vi "MultiPlotting_6PlotForADC.vi"(0 "2D-DataIn":dbl[][](array[numeric]), 3 "DisplayControl":T2 {"Scale" items=["L", "R"]; "Y - axes"."Y 6" items=["", "Realtime_sec", "Intervaltime_sec", "OscillatorFreq_Hz", "SR7265_1_Vx_Volt", "SR7265_1_Vy_Volt", "Ohm"]; "Y - axes"."Y 5" items=["", "Realtime_sec", "Intervaltime_sec", "OscillatorFreq_Hz", "SR7265_1_Vx_Volt", "SR7265_1_Vy_Volt", "Ohm"]; "Y - axes"."Y 4" items=["", "Realtime_sec", "Intervaltime_sec", "OscillatorFreq_Hz", "SR7265_1_Vx_Volt", "SR7265_1_Vy_Volt", "Ohm"]; "Y - axes"."Y 3" items=["", "Realtime_sec", "Intervaltime_sec", "OscillatorFreq_Hz", "SR7265_1_Vx_Volt", "SR7265_1_Vy_Volt", "Ohm"]; "Y - axes"."Y 2" items=["", "Realtime_sec", "Intervaltime_sec", "OscillatorFreq_Hz", "SR7265_1_Vx_Volt", "SR7265_1_Vy_Volt", "Ohm"]; "Y - axes"."Y 1" items=["", "Realtime_sec", "Intervaltime_sec", "OscillatorFreq_Hz", "SR7265_1_Vx_Volt", "SR7265_1_Vy_Volt", "Ohm"]; "X - axis" items=["Realtime_sec", "Intervaltime_sec", "OscillatorFreq_Hz", "SR7265_1_Vx_Volt", "SR7265_1_Vy_Volt", "Ohm"]}) -> (5 "DataDisplay":T1 {"X" format="%#_6e"; "Y 5" format="%#_6e"; "Y 4" format="%#_6e"; "Y 3" format="%#_6e"; "Y 6" format="%#_6e"; "Y 2" format="%#_6e"; "Y 1" format="%#_6e"}, 7 "XY Graph":cluster{"DataOut":dbl[], "DataOut":dbl[]}[](graph))   [LabVIEW 2012]
doc: "2D array input, and select 6 colums to plot XY graph. This subVI only support 6 plotting lines. If more than 6 plottings are required, please increase the number of Y-axes control ring in DisplayControl."
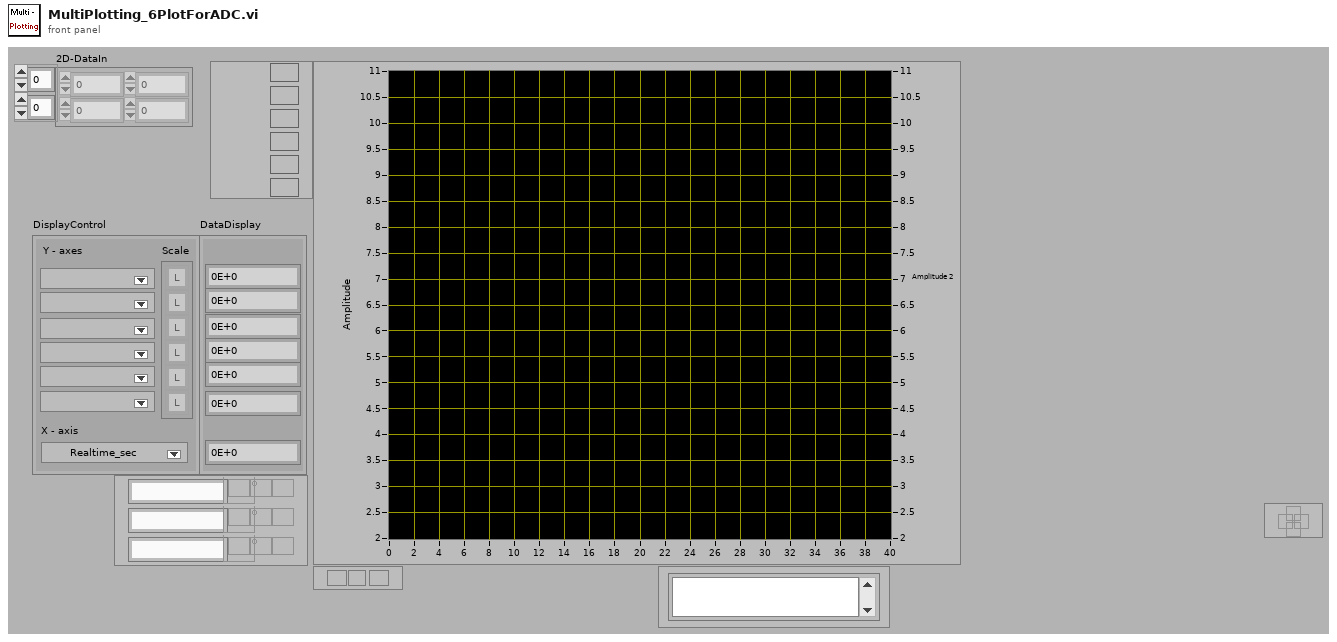
[diagram p1: front panel]
types:
  T1 = cluster{"X":dbl, "Y 1":dbl, "Y 2":dbl, "Y 3":dbl, "Y 4":dbl, "Y 5":dbl, "Y 6":dbl}
  T2 = cluster{"X - axis":u8, "Y - axes":cluster{"Y 1":u8, "Y 2":u8, "Y 3":u8, "Y 4":u8, "Y 5":u8, "Y 6":u8}, "Scale":u16[]}
  T3 = cluster{"Y 1":u8, "Y 2":u8, "Y 3":u8, "Y 4":u8, "Y 5":u8, "Y 6":u8}
  T4 = cluster{"[0]":dbl, "[1]":dbl, "[2]":dbl, "[3]":dbl, "[4]":dbl, "[5]":dbl, "[6]":dbl}
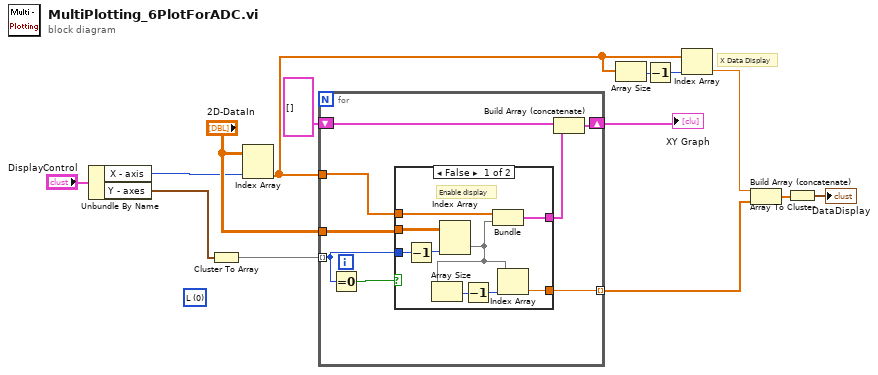
[diagram p0: block diagram]
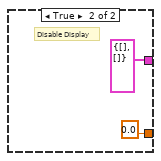
[diagram p2: hidden frame]
diagram:
  (unwired) u16 0 items=["L", "R"] ("Y-axes slector 2")
  # "X Data Display"
  n1 = Unbundle By Name("DisplayControl") -> ("X - axis"=w11:u8, "Y - axes"=w13:T3)
  n2 = Cluster To Array(cluster=w13) -> (array=w14:u8[])
  n3 = Index Array(array="2D-DataIn", index (col)=w11) -> (element=w5:dbl[])  [unwired: 1 in]
  n4 = for {
    tunnel: w14 -> [w18] mode=indexing
    shift-right: [w21] -> w9
    shift-left: cluster{"DataOut":dbl[], "DataOut":dbl[]}[] [] -> [w20]
    tunnel: w5 -> [w17]
    tunnel: "2D-DataIn" -> [w19]
    tunnel: [w16] -> w3 mode=indexing
    n5 = Equal To 0?(x=w18) -> (x = 0?=w15:bool)
    n6 = case shown="False" w15 {
      tunnel: w19 -> [w31 _]
      tunnel: w17 -> [w30 _]
      tunnel: [w29 cluster{"DataOut":dbl[], "DataOut":dbl[]} {"DataOut"=[], "DataOut"=[]}] -> w22
      tunnel: w18 -> [w28 _]
      tunnel: [w23 0.0] -> w16
      frame False {
        # "Enable display"
        n7 = Decrement(x=w28) -> (x-1=w27:u8)
        n8 = Index Array(array=w31, index (col)=w27) -> (element=w24:dbl[])  [unwired: 1 in]
        n9 = Array Size(array=w24) -> (size(s)=w25:i32)
        n10 = Decrement(x=w25) -> (x-1=w26:i32)
        n11 = Bundle("2D-DataIn"=w30, "2D-DataIn"=w24) -> (w29:cluster{"2D-DataIn":dbl[], "2D-DataIn":dbl[]})  [unwired: 1 out]
        n12 = Index Array(array=w24, index=w26) -> (element=w23:dbl)
      }
      frame True {
        # "Disable Display"
      }
    }
    n13 = Build Array (concatenate)(w20, w22) -> (w21:cluster{"DataOut":dbl[], "DataOut":dbl[]}[])
  }
  "XY Graph" <- w9
  n14 = Array Size(array=w5) -> (size(s)=w6:i32)
  n15 = Decrement(x=w6) -> (x-1=w7:i32)
  n16 = Index Array(array=w5, index=w7) -> (element=w4:dbl)
  n17 = Build Array (concatenate)(w4, w3) -> (w2:dbl[])
  n18 = Array To Cluster(array=w2) -> (cluster=→"DataDisplay":T4)
